vi "Gear Shift Timer.vi"(0 "In 1":dbl, 1 "In 2":dbl, 2 "In 3":dbl, 3 "In 4":dbl, 6 "1st Gear?":bool, 8 "RESET THE CLOCKS":bool) -> (11 "2nd Gear Shifts":dbl, 13 "1st Gear Shifts":dbl, 14 "Out 1":dbl, 15 "Out 2":dbl, 16 "Out 3":dbl, 17 "Out 4":dbl, 18 "1st Gear Time":dbl, 19 "2nd Gear Time":dbl)   [LabVIEW 2015]
uses:
  Common Code/Change Detect Boolean.vi
panel:
  in  "Saved Time 2":dbl
  in  "Saved Time 1":dbl
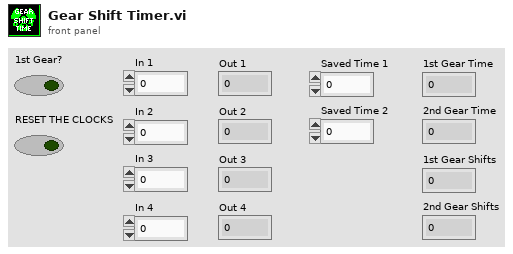
[diagram p1: front panel]
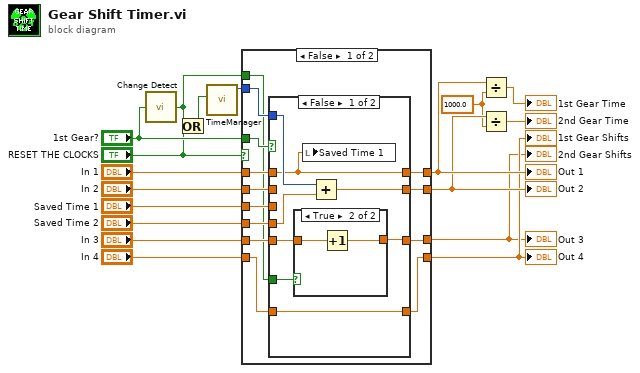
[diagram p0: block diagram]
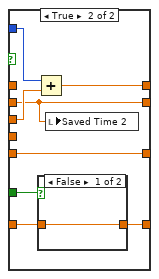
[diagram p3: hidden frame]
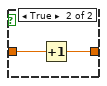
[diagram p4: hidden frame]
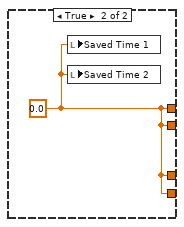
[diagram p5: hidden frame]
diagram:
  w3 = 1000.0 ("y")
  n1 = call-poly "Change Detect.vi"("In"="1st Gear?") -> ("Changed?"=w7:bool)
  n2 = Or(x=w7, y="RESET THE CLOCKS") -> (x .or. y?=w5:bool)
  n3 = call "TimeManager.vi"("Reset?"=w5) -> ("Time Since Reset"=w18:u32)  [unwired: 9 in, 1 out]
  n4 = case shown="False" "RESET THE CLOCKS" {
    tunnel: w18 -> [w30 _]
    tunnel: "1st Gear?" -> [w31 _]
    tunnel: "In 1" -> [w24 _]
    tunnel: "In 2" -> [w27 _]
    tunnel: "In 3" -> [w23 _]
    tunnel: "In 4" -> [w20 _]
    tunnel: [w28 w54] -> w12
    tunnel: [w26 w54] -> w4
    tunnel: [w22 w54] -> w1
    tunnel: [w19 w54] -> w2
    tunnel: "Saved Time 1" -> [w29 _]
    tunnel: "Saved Time 2" -> [w25 _]
    tunnel: w7 -> [w21 _]
    frame False {
      n5 = case shown="False" w31 {
        tunnel: w30 -> [w39 w49]
        tunnel: w29 -> [_ w50]
        tunnel: [w36 w48] -> w28
        tunnel: w27 -> [_ w47]
        tunnel: [w37 w47] -> w26
        tunnel: w25 -> [w38 _]
        tunnel: w24 -> [w36 _]
        tunnel: w23 -> [w33 w46]
        tunnel: [w32 w46] -> w22
        tunnel: w21 -> [w34 w45]
        tunnel: w20 -> [w35 w44]
        tunnel: [w35 w43] -> w19
        frame False {
          n6 = case shown="True" w34 {
            tunnel: w33 -> [w40 w42]
            tunnel: [w40 w41] -> w32
            frame False {
            }
            frame True {
              n7 = Increment(x=w42) -> (x+1=w41:dbl)
            }
          }
          n8 = local write "Saved Time 1"(w36) -> ()
          n9 = Add(x=w39, y=w38) -> (x+y=w37:dbl)
        }
        frame True {
          n10 = Add(x=w49, y=w50) -> (x+y=w48:dbl)
          n11 = case shown="False" w45 {
            tunnel: w44 -> [w51 w53]
            tunnel: [w51 w52] -> w43
            frame False {
            }
            frame True {
              n12 = Increment(x=w53) -> (x+1=w52:dbl)
            }
          }
          n13 = local write "Saved Time 2"(w47) -> ()
        }
      }
    }
    frame True {
      w54 = 0.0
      n14 = local write "Saved Time 1"(w54) -> ()
      n15 = local write "Saved Time 2"(w54) -> ()
    }
  }
  "Out 1" <- w12
  "Out 2" <- w4
  "Out 3" <- w1
  "Out 4" <- w2
  "1st Gear Shifts" <- w2
  "2nd Gear Shifts" <- w1
  n16 = Divide(x=w12, y=w3) -> (x/y=→"1st Gear Time":dbl)
  n17 = Divide(x=w4, y=w3) -> (x/y=→"2nd Gear Time":dbl)
